vi "数据插入.vi"(5 "数据标记表":string(combo)="N", 7 "测量模式":string(combo), 8 "error in (no error)":errorcluster caption="错误输入（无错误）", 10 "data in":T1={"因子编码"="", "单位"="", "标样参考值"=0.0, "水样数据时间"=timestamp(0 s since 1904-01-01), "水样实测值"=0.0, "水样数据标识"="N", "探头温度"=0.0}, 11 "table输入":string(combo)) -> (0 "error out":errorcluster caption="错误输出")   [LabVIEW 2016, in "斯坦道多参数.lvlib"]
uses:
  <vilib>/Utility/sysdir.llb/System Directory Type.ctl
  <vilib>/Utility/error.llb/DialogType.ctl
  <vilib>/addons/database/Connection.llb/DB Tools Open Connec (String).vi
  <vilib>/addons/database/Connection.llb/Conn Execute.vi
  <vilib>/addons/database/Recordset.llb/Rec Destroy - Connection.vi
  <vilib>/addons/database/NI_Database_API.lvlib
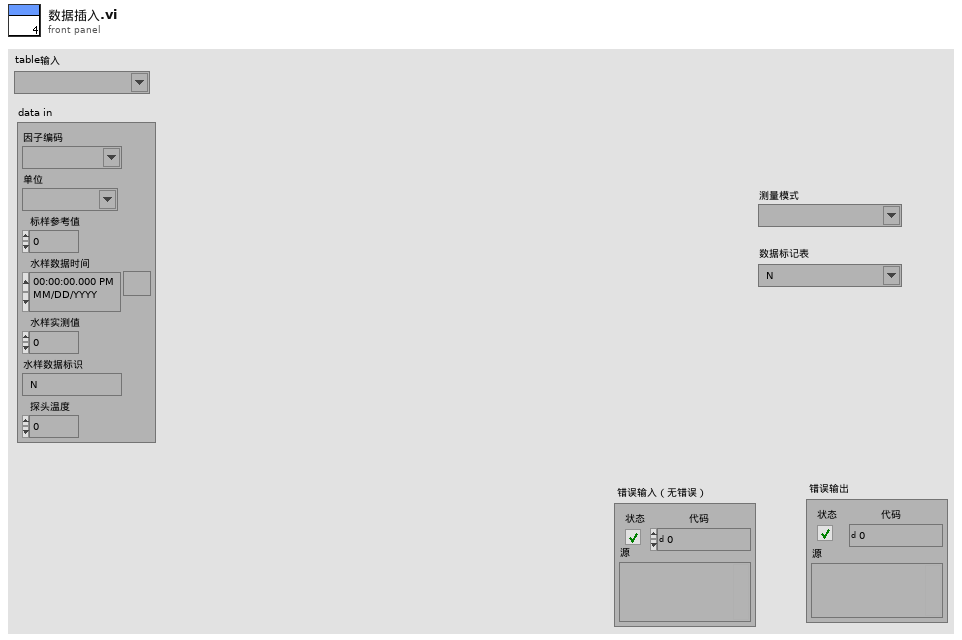
[diagram p1: front panel]
types:
  T1 = cluster{"因子编码":string, "单位":string, "标样参考值":sgl, "水样数据时间":timestamp, "水样实测值":sgl, "水样数据标识":string, "探头温度":sgl}
  T2 = typedef "DialogType.ctl" = u16
  T3 = typedef "System Directory Type.ctl" = i32
  T4 = cluster{"时间标识":timestamp, "测量模式":string, "数据类型":string, "监测值":sgl, "单位":string, "数据标识":string, "因子编码":string, "标样参考值":sgl, "探头温度":sgl, "LastTime":timestamp}
  T5 = typedef "NI_Database_API.lvlib/Conn ObjectReference.ctl" = refnum<k1>
  T6 = typedef "NI_Database_API.lvlib/Rec ObjectReference.ctl" = refnum<k1>
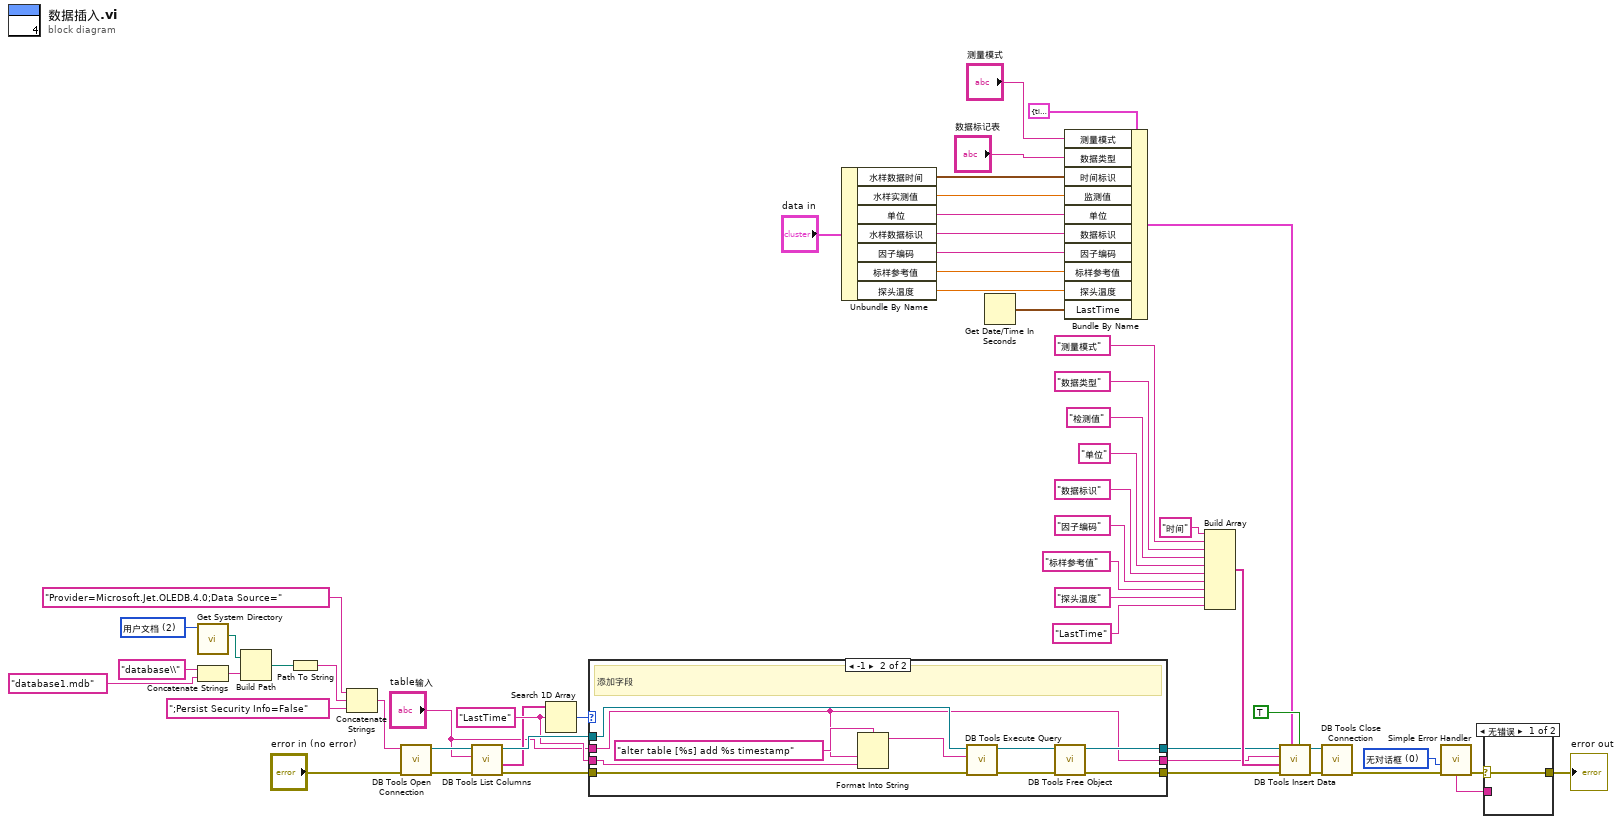
[diagram p0: block diagram]
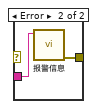
[diagram p2: hidden frame]
diagram:
  w4 = T2 0 items=["无对话框", "确定信息", "继续或停止信息", "确定信息＋警告", "继续/停止+警告"] ("type of dialog (OK msg:1)")
  w16 = "LastTime" ("元素")
  w35 = T3 2 items=["用户目录"=0, "用户桌面"=1, "用户文档"=2, "用户应用程序数据"=3, "用户设置"=4, "用户临时目录"=5, "公共文档"=6, "公共应用程序数据"=7, "公共设置"=8, "公共缓存"=13, "系统核心库"=9, "系统安装库"=10, "应用程序文件"=11, "启动盘根目录"=12] ("system directory type")
  n1 = call <vilib>:"Get System Directory.vi"("system directory type"=w35) -> ("system directory"=w33:path)  [unwired: 10 in]
  n2 = Concatenate Strings("database\\" ("condition"), "database1.mdb" ("字符串")) -> (w27:string)
  n3 = Build Path(base path=w33, name or relative path=w27) -> (appended path=w32:path)
  n4 = Path To String(path=w32) -> (string=w31:string)
  n5 = Concatenate Strings("Provider=Microsoft.Jet.OLEDB.4.0;Data Source=" ("condition"), w31, ";Persist Security Info=False" ("condition")) -> (w29:string)
  n6 = call-poly <vilib>:"DB Tools Open Connection.vi"("error in (no error)"="error in (no error)", "connection information"=w29) -> ("error out"=w18:errorcluster, "connection reference"=w19:T5)  [unwired: 6 in]
  n7 = call <vilib>:"DB Tools List Columns.vi"("error in (no error)"=w18, "table"="table输入", "connection reference"=w19) -> ("error out"=w14:errorcluster, "columns"=w15:string[], "connection reference out"=w17:T5)  [unwired: 1 in, 1 out]
  n8 = Search 1D Array(1D array=w15, element=w16) -> (index of element=w13:i32)  [unwired: 1 in]
  n9 = case shown="-1" w13 {
    tunnel: w17 -> [w57 w65]
    tunnel: w14 -> [w56 w64]
    tunnel: w16 -> [_ w62]
    tunnel: [w57 w60] -> w12
    tunnel: [w56 w59] -> w11
    tunnel: "table输入" -> [w55 w58]
    tunnel: [w55 w58] -> w9
    frame 0, Default {
    }
    frame -1 {
      # "添加字段"
      n10 = Format Into String(format string="alter table [%s] add %s timestamp", w58, w62) -> (resulting string=w61:string)  [unwired: 2 in, 1 out]
      n11 = call-poly <vilib>:"DB Tools Execute Query.vi"("error in (no error)"=w64, "SQL query"=w61, "connection reference"=w65) -> ("error out"=w66:errorcluster, "recordset reference"=w67:T6)  [unwired: 5 in]
      n12 = call-poly <vilib>:"DB Tools Free Object.vi"("error in (no error)"=w66, "recordset reference"=w67) -> ("error out"=w59:errorcluster, "connection reference"=w60:T5)  [unwired: 8 in]
    }
  }
  n13 = Unbundle By Name("data in") -> ("水样数据时间"=w49:timestamp, "水样实测值"=w48:sgl, "单位"=w44:string, "水样数据标识"=w47:string, "因子编码"=w43:string, "标样参考值"=w45:sgl, "探头温度"=w24:sgl)
  n14 = Get Date/Time In Seconds() -> (seconds since 1Jan1904=w7:timestamp)
  n15 = Bundle By Name(cluster=T4 {"时间标识"=timestamp(0 s since 1904-01-01), "测量模式"="", "数据类型"="", "监测值"=0.0, "单位"="", "数据标识"="", "因子编码"="", "标样参考值"=0.0, "探头温度"=0.0, "LastTime"=timestamp(0 s since 1904-01-01)} ("data输出"), "测量模式"="测量模式", "数据类型"="数据标记表", "时间标识"=w49, "监测值"=w48, "单位"=w44, "数据标识"=w47, "因子编码"=w43, "标样参考值"=w45, "探头温度"=w24, "LastTime"=w7) -> (w25:T4)
  n16 = Build Array("时间", "测量模式", "数据类型", "检测值", "单位", "数据标识", "因子编码", "标样参考值", "探头温度", "LastTime") -> (w26:string[])
  n17 = call <vilib>:"DB Tools Insert Data.vi"("create table? (F)"=TRUE, "data"=w25, "error in (no error)"=w11, "columns"=w26, "table"=w9, "connection reference"=w12) -> ("error out"=w37:errorcluster, "connection reference out"=w38:T5)  [unwired: 4 in]
  n18 = call <vilib>:"DB Tools Close Connection.vi"("error in (no error)"=w37, "connection reference"=w38) -> ("error out"=w5:errorcluster)  [unwired: 5 in]
  n19 = call <vilib>:"Simple Error Handler.vi"("type of dialog (OK msg:1)"=w4, "error in (no error)"=w5) -> ("error out"=w2:errorcluster, "message"=w3:string)  [unwired: 3 in, 3 out]
  n20 = case shown="无错误" w2 {
    selector: w2 -> [w68 _]
    tunnel: w3 -> [_ w70]
    tunnel: [w68 w69] -> w1
    frame No Error {
    }
    frame Error {
      n21 = call "报警信息.vi"("报警信息"=w70) -> ("error out"=w69:errorcluster)  [unwired: 10 in]
    }
  }
  "error out" <- w1
